vi "Testing - Go To Position.vi"() -> ()   [LabVIEW 2015]
uses:
  Position.ctl
  Type Defs/Direction Enum.ctl
  Square/Board Size.vi
  SubVIs/Read-Only Globals.vi
  SubVIs/Globals (private).vi
  Common.lvlib
  Type Defs/SB Type Defs.lvlib
panel:
  out "Arrived?":bool
  out "Direction":T1
  out "Position out":T2
  in  "Target Position":T2
  in  "My Position":T2
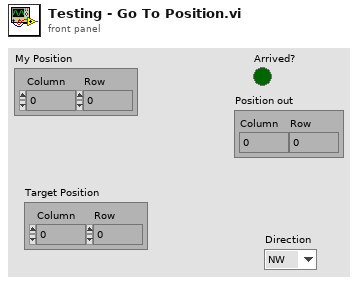
[diagram p1: front panel]
types:
  T1 = typedef "SB Type Defs.lvlib/Direction Enum.ctl" = enum16{"NW", "N", "NE", "E", "SE", "S", "SW", "W"}
  T2 = typedef "Common.lvlib/Position.ctl" = cluster{"Column":i32, "Row":i32}
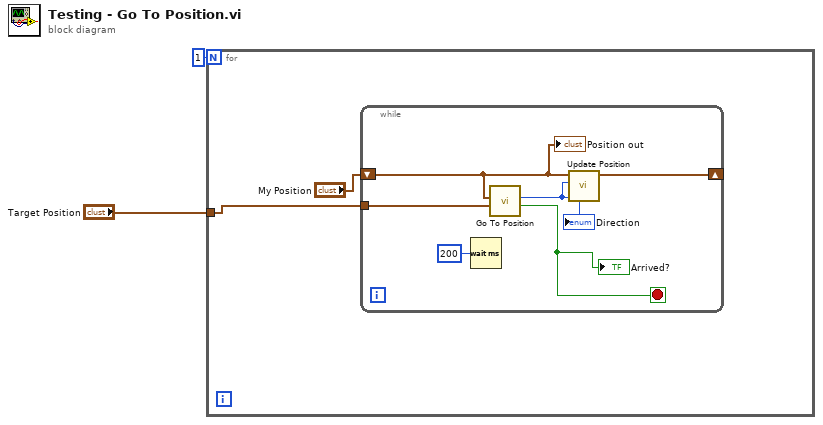
[diagram p0: block diagram]
diagram:
  n1 = for {
    N: 1 -> [_]
    tunnel: "Target Position" -> [w3]
    n2 = while {
      shift-right: [w10] -> _
      shift-left: "My Position" -> [w6]
      tunnel: w3 -> [w9]
      stop <- w5 stop-if-true
      n3 = Wait (ms)(milliseconds to wait=u32 200) -> ()  [unwired: 1 out]
      n4 = call "Go To Position.vi"("Target Position"=w9, "My Position"=w6) -> ("Arrived?"=w5:bool, "Direction"=w8:T1)  [unwired: 7 in, 1 out]
      "Direction" <- w8
      "Arrived?" <- w5
      n5 = call "Update Position.vi"("Direction"=w8, "Position in"=w6) -> ("Position out"=w10:T2)  [unwired: 9 in]
      "Position out" <- w6
    }
  }
